vi "LR-Find-edges.vi"(7 "Sample divide settings":T2={"Accept only complete pulses"=TRUE, "Edge treshold [%]"=15}, 8 "error in (no error)":errorcluster, 10 "Control in":u32[](array[numeric]), 11 "Results in":T1) -> (0 "error out":errorcluster, 2 "Control":u32[](array[numeric]), 3 "Results":T1, 4 "Valid?":bool)   [LabVIEW 2013, in "MaterialCharacterization.lvlib" / "MC-LaserResponse.lvclass"]
doc: "Use this template to build a VI to use as a subVI."
uses:
  MC-LaserResponse.lvclass
  Settings-divide.ctl
  Test-results.ctl
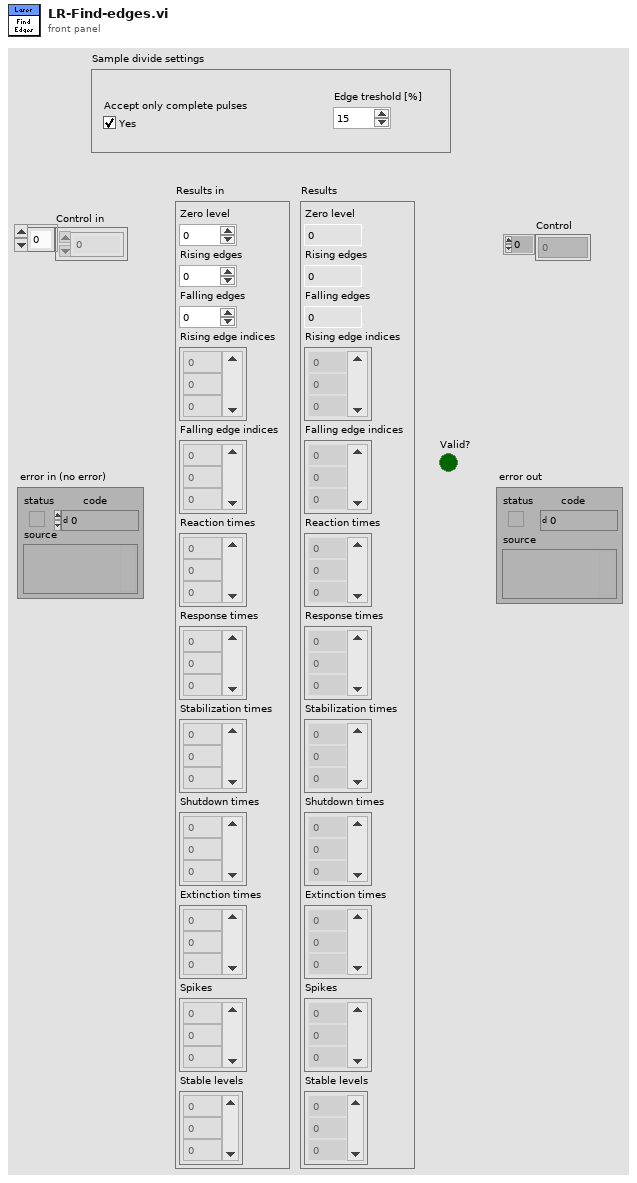
[diagram p1: front panel]
types:
  T1 = typedef "MaterialCharacterization.lvlib/MC-LaserResponse.lvclass/Test-results.ctl" = cluster{"Zero level":dbl, "Rising edges":i32, "Falling edges":i32, "Rising edge indices":dbl[], "Falling edge indices":dbl[], "Reaction times":dbl[], "Response times":dbl[], "Stabilization times":dbl[], "Shutdown times":dbl[], "Extinction times":dbl[], "Spikes":i32[], "Stable levels":dbl[]}
  T2 = typedef "MaterialCharacterization.lvlib/MC-LaserResponse.lvclass/Settings-divide.ctl" = cluster{"Accept only complete pulses":bool, "Edge treshold [%]":i32}
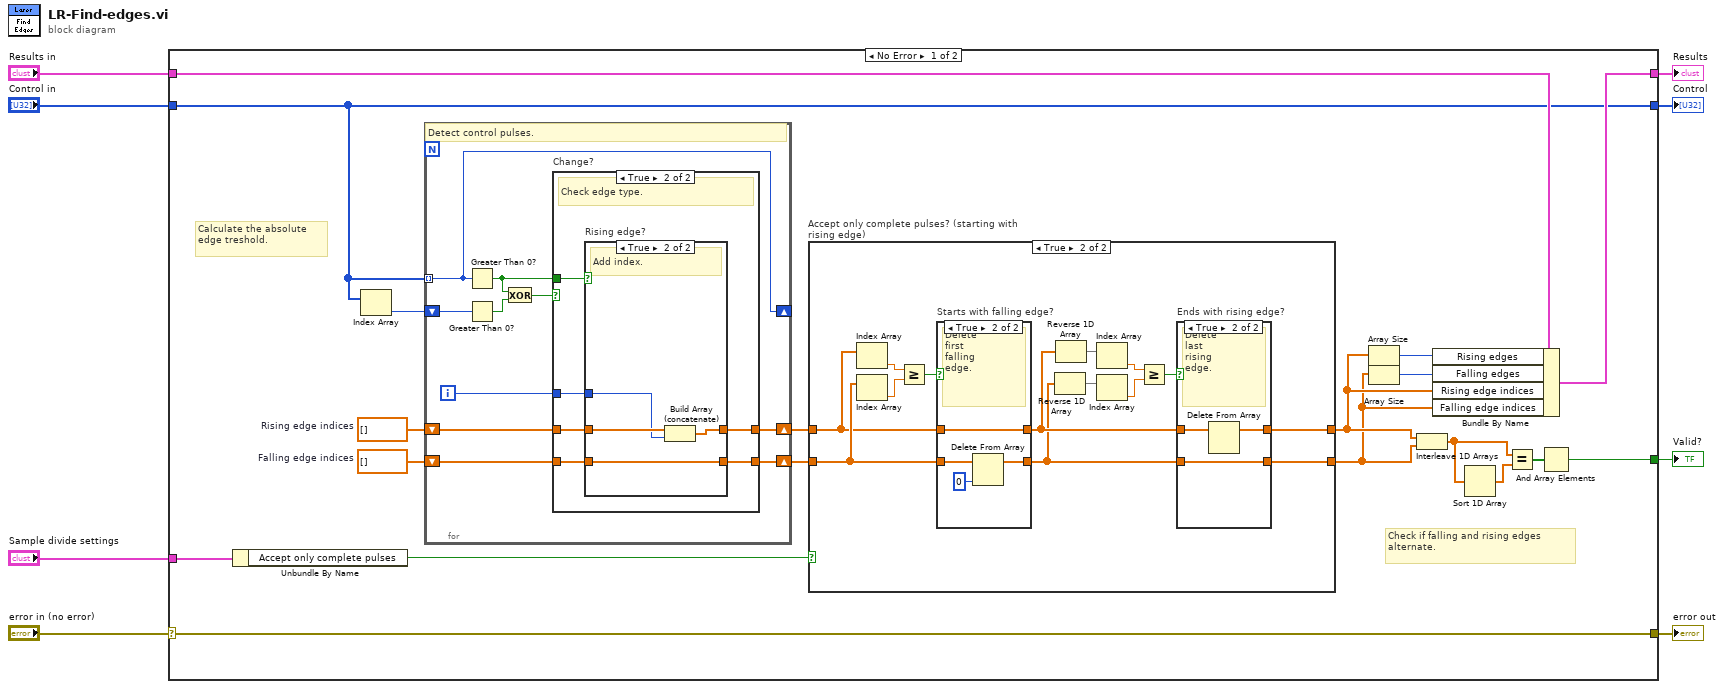
[diagram p0: block diagram]
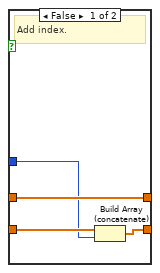
[diagram p6: hidden frame]
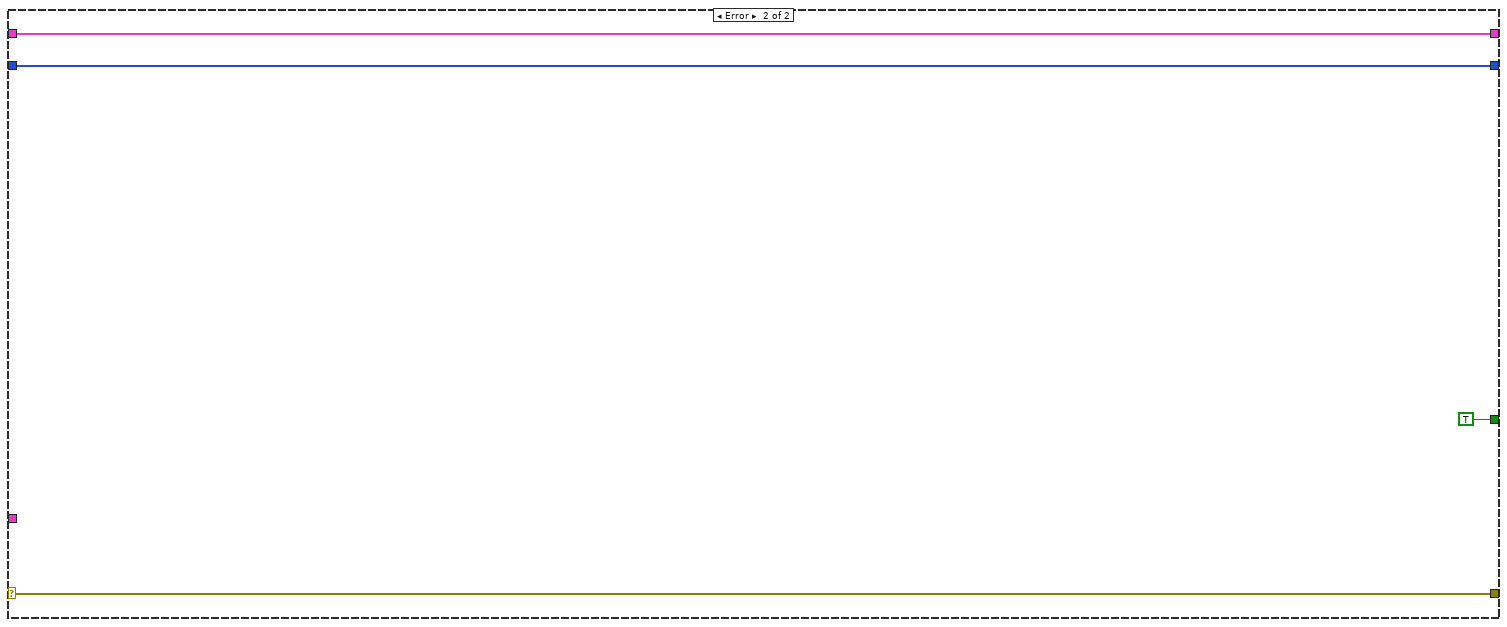
[diagram p7: hidden frame]
diagram:
  n1 = case shown="No Error" "error in (no error)" {
    selector: "error in (no error)" -> [w23 w84]
    tunnel: [w23 w84] -> w7
    tunnel: "Results in" -> [w10 w83]
    tunnel: "Sample divide settings" -> [w27 _]
    tunnel: [w17 TRUE] -> w5
    tunnel: [w16 w83] -> w2
    tunnel: "Control in" -> [w9 w81]
    tunnel: [w9 w81] -> w1
    frame No Error {
      w25 = dbl[] []  # Falling edge indices
      w24 = dbl[] []  # Rising edge indices
      # "Calculate the absolute\nedge treshold."
      # "Check if falling and rising edges\nalternate."
      n2 = Unbundle By Name(w27) -> ("Accept only complete pulses"=w13:bool)
      n3 = Index Array(array=w9) -> (element=w26:u32)  [unwired: 1 in]
      n4 = for {
        tunnel: w9 -> [w57] mode=indexing
        shift-right: [w58] -> w15
        shift-left: w24 -> [w61]
        shift-right: [w59] -> w14
        shift-left: w25 -> [w60]
        shift-right: [w57] -> _
        shift-left: w26 -> [w56]
        i -> [w55]
        # "Detect control pulses."
        n5 = Greater Than 0?(x=w57) -> (x > 0?=w62:bool)
        n6 = Greater Than 0?(x=w56) -> (x > 0?=w63:bool)
        n7 = Exclusive Or(1:w63, 2:w62) -> (0:w64:bool)
        n8 = case "Change?" shown="True" w64 {
          tunnel: w62 -> [_ w72]
          tunnel: w61 -> [w66 w71]
          tunnel: w60 -> [w65 w70]
          tunnel: w55 -> [_ w69]
          tunnel: [w65 w68] -> w59
          tunnel: [w66 w67] -> w58
          frame False {
            # "Do nothing."
          }
          frame True {
            # "Check edge type."
            n9 = case "Rising edge?" shown="True" w72 {
              tunnel: w71 -> [w74 w79]
              tunnel: w70 -> [w76 w80]
              tunnel: w69 -> [w73 w77]
              tunnel: [w75 w80] -> w68
              tunnel: [w74 w78] -> w67
              frame False {
                # "Add index."
                n10 = Build Array (concatenate)(w76, w73) -> (w75:dbl[])
              }
              frame True {
                # "Add index."
                n11 = Build Array (concatenate)(w79, w77) -> (w78:dbl[])
              }
            }
          }
        }
      }
      n12 = case "Accept only complete pulses? (starting with rising edge)" shown="True" w13 {
        tunnel: w15 -> [w29 w39]
        tunnel: w14 -> [w28 w41]
        tunnel: [w29 w31] -> w12
        tunnel: [w28 w30] -> w11
        frame False {
        }
        frame True {
          n13 = Index Array(array=w39) -> (element=w43:dbl)  [unwired: 1 in]
          n14 = Index Array(array=w41) -> (element=w42:dbl)  [unwired: 1 in]
          n15 = Greater Or Equal?(x=w43, y=w42) -> (x >= y?=w40:bool)
          n16 = case "Starts with falling edge?" shown="True" w40 {
            tunnel: w41 -> [w49 w54]
            tunnel: w39 -> [w50 w52]
            tunnel: [w50 w52] -> w35
            tunnel: [w49 w51] -> w34
            frame False {
            }
            frame True {
              # "Delete\nfirst\nfalling\nedge."
              n17 = Delete From Array(array=w54, index=0) -> (array with subset deleted=w51:dbl[])  [unwired: 1 in, 1 out]
            }
          }
          n18 = Reverse 1D Array(array=w34) -> (reversed array=w32:dbl[])
          n19 = Reverse 1D Array(array=w35) -> (reversed array=w33:dbl[])
          n20 = Index Array(array=w33) -> (element=w36:dbl)  [unwired: 1 in]
          n21 = Index Array(array=w32) -> (element=w37:dbl)  [unwired: 1 in]
          n22 = Greater Or Equal?(x=w36, y=w37) -> (x >= y?=w38:bool)
          n23 = case "Ends with rising edge?" shown="True" w38 {
            tunnel: w34 -> [w44 w46]
            tunnel: w35 -> [w45 w48]
            tunnel: [w45 w47] -> w31
            tunnel: [w44 w46] -> w30
            frame False {
            }
            frame True {
              # "Delete\nlast\nrising\nedge."
              n24 = Delete From Array(array=w48) -> (array with subset deleted=w47:dbl[])  [unwired: 2 in, 1 out]
            }
          }
        }
      }
      n25 = Array Size(array=w12) -> (size(s)=w22:i32)
      n26 = Array Size(array=w11) -> (size(s)=w21:i32)
      n27 = Interleave 1D Arrays(w12, w11) -> (w20:dbl[])
      n28 = Bundle By Name(cluster=w10, "Rising edges"=w22, "Falling edges"=w21, "Rising edge indices"=w12, "Falling edge indices"=w11) -> (w16:T1)
      n29 = Sort 1D Array(array=w20) -> (sorted array=w19:dbl[])
      n30 = Equal?(x=w20, y=w19) -> (x = y?=w18:bool[])
      n31 = And Array Elements(Boolean array=w18) -> (logical AND=w17:bool)
    }
    frame Error {
    }
  }
  "error out" <- w7
  "Valid?" <- w5
  "Results" <- w2
  "Control" <- w1
